vi "Create and Queue New Plugin Command.vi"(8 "error in (no error)":errorcluster, 9 "Matching Plugin":T1, 10 "New Plugin":T5, 11 "CIFPluginManager in":refnum<class "CIFPluginManager.lvclass">) -> (0 "error out":errorcluster)   [LabVIEW 2021, in "CIFPluginManager.lvclass"]
uses:
  CIFPluginManager.lvclass
  typedef/Plugin Load Command.ctl
  typedef/Loader Type.ctl
  typedef/Discovered Plugin.ctl
  <vilib>/CIF Foundation/CIF Core/CIFCore/Common/Typedef/Version.ctl
  typedef/Plugin Metadata.ctl
  CIFPluginManager.lvclass/CIFPluginManager.ctl
  typedef/Plugin Management Data.ctl
  <vilib>/gRPC/LabVIEW gRPC Library/Shared/grpcId.ctl
  gRPC/CIF_Manager_server/RPC Messages/cif_management_common_PluginStatusData.ctl
  gRPC/CIF_Manager_server/RPC Messages/cif_management_common_PluginStatusData_PluginState.ctl
  gRPC/CIF_Manager_server/RPC Messages/cif_management_common_TimingStatistics.ctl
  gRPC/CIF_Manager_server/RPC Messages/cif_common_TimingStats.ctl
  gRPC/CIF_Manager_server/RPC Messages/cif_management_common_FifoStatistics.ctl
  gRPC/CIF_Manager_server/RPC Messages/cif_management_common_Error.ctl
  gRPC/CIF_Manager_server/RPC Messages/cif_management_common_MonitorDoubles.ctl
  gRPC/CIF_Manager_server/RPC Messages/cif_management_common_MonitorU64.ctl
  gRPC/CIF_Manager_server/RPC Messages/cif_management_common_MonitorI64.ctl
  gRPC/CIF_Manager_server/RPC Messages/cif_management_common_Channels.ctl
  gRPC/CIF_Manager_server/RPC Messages/cif_management_common_Channel.ctl
  gRPC/CIF_Manager_server/RPC Messages/cif_management_common_ChannelDirection.ctl
  gRPC/CIF_Manager_server/RPC Messages/cif_management_common_ChannelPattern.ctl
  gRPC/CIF_Manager_server/CIF_Manager_server.lvlib
  <vilib>/CIF Foundation/CIF Core/CIFCore/Common/CIFCoreCommon.lvlib
  <vilib>/gRPC/LabVIEW gRPC Library/grpc-lvsupport-release.lvlib
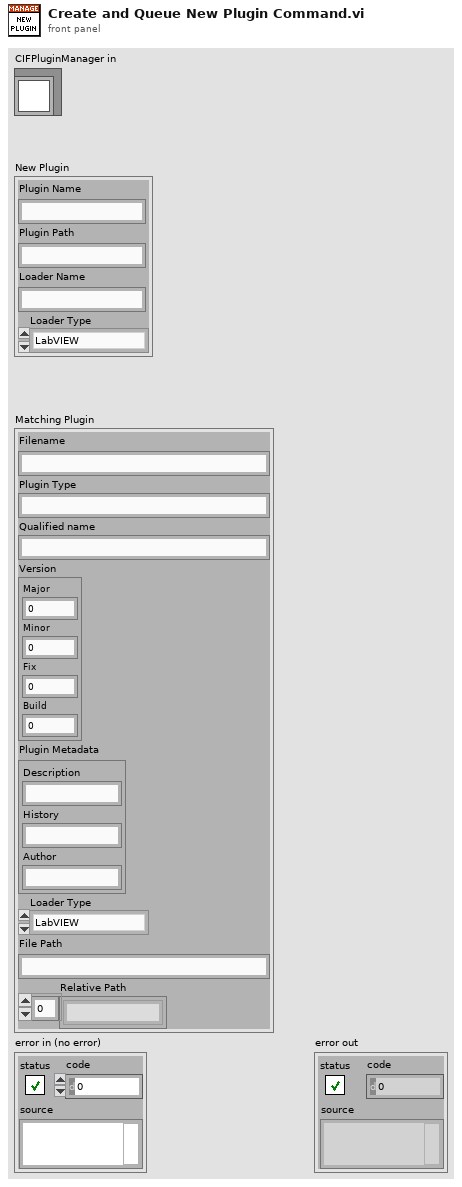
[diagram p1: front panel]
types:
  T1 = typedef "CIFPluginManager.lvclass/Discovered Plugin.ctl" = cluster{"Filename":string, "Plugin Type":string, "Qualified name":string, "Version":T2, "Plugin Metadata":T3, "Loader Type":T4, "File Path":string, "Relative Path":string[]}
  T2 = typedef "CIFCoreCommon.lvlib/Version.ctl" = cluster{"Major":i32, "Minor":i32, "Fix":i32, "Build":i32}
  T3 = typedef "CIFPluginManager.lvclass/Plugin Metadata.ctl" = cluster{"Description":string, "History":string, "Author":string}
  T4 = typedef "CIFPluginManager.lvclass/Loader Type.ctl" = enum16{"LabVIEW"}
  T5 = typedef "CIFPluginManager.lvclass/Plugin Load Command.ctl" = cluster{"Plugin Name":string, "Plugin Path":string, "Loader Name":string, "Loader Type":T4}
  T6 = typedef "CIFPluginManager.lvclass/Loader Map.ctl" = map{string, T7}
  T7 = typedef "CIFPluginManager.lvclass/Loaders.ctl" = cluster{"Loader Type":T4, "grpc_port":i32, "pid":u32, "gRPC ID":T8, "Load Timestamp":i64, "Unloading":bool, "Ready for removal":bool, "Unload Timestamp":i64}
  T8 = typedef "grpc-lvsupport-release.lvlib/grpcId.ctl" = u64
  T9 = typedef "CIFPluginManager.lvclass/Plugin Management Data.ctl" = cluster{"Unique Name":string, "Plugin Type":string, "gRPC Port":i32, "gRPC ID":T8, "Loader Type":T4, "Loader":string, "Version":T2, "Load Timestamp":i64, "Unload Timestamp":i64, "Unloading":bool, "Ready for removal":bool, "status":T10, "channels":T19}
  T10 = typedef "CIF_Manager_server.lvlib/cif_management_common_PluginStatusData.ctl" = cluster{"state":T11, "timing_statistics":T12, "fifo_statistics":T14, "error":T15, "monitor_doubles":T16, "monitor_u64s":T17, "monitor_i64s":T18}
  T11 = typedef "CIF_Manager_server.lvlib/cif_management_common_PluginStatusData_PluginState.ctl" = enum32{"PLUGINSTATE_UNKNOWN", "PLUGINSTATE_CREATING", "PLUGINSTATE_LISTENING", "PLUGINSTATE_RUNNING", "PLUGINSTATE_CLEANINGUP", "PLUGINSTATE_DESTROYING"}
  T12 = typedef "CIF_Manager_server.lvlib/cif_management_common_TimingStatistics.ctl" = cluster{"period":T13, "wake_error":T13, "execute":T13, "housekeep":T13, "idle":T13, "cleanup":T13, "custom_1":T13, "custom_2":T13}
  T13 = typedef "CIF_Manager_server.lvlib/cif_common_TimingStats.ctl" = cluster{"max":i64, "min":i64, "avg":dbl}
  T14 = typedef "CIF_Manager_server.lvlib/cif_management_common_FifoStatistics.ctl" = cluster{"from_t0":T13, "from_previous_plugin":T13, "output_error":T13}
  T15 = typedef "CIF_Manager_server.lvlib/cif_management_common_Error.ctl" = cluster{"status":bool, "code":i32}
  T16 = typedef "CIF_Manager_server.lvlib/cif_management_common_MonitorDoubles.ctl" = cluster{"double_1":dbl, "double_2":dbl, "double_3":dbl, "double_4":dbl}
  T17 = typedef "CIF_Manager_server.lvlib/cif_management_common_MonitorU64.ctl" = cluster{"u64_1":u64, "u64_2":u64, "u64_3":u64, "u64_4":u64}
  T18 = typedef "CIF_Manager_server.lvlib/cif_management_common_MonitorI64.ctl" = cluster{"i64_1":i64, "i64_2":i64, "i64_3":i64, "i64_4":i64}
  T19 = typedef "CIF_Manager_server.lvlib/cif_management_common_Channels.ctl" = cluster{"channels":T20[]}
  T20 = typedef "CIF_Manager_server.lvlib/cif_management_common_Channel.ctl" = cluster{"name":string, "direction":T21, "type":string, "custom_config":u8[], "connected":bool, "connected_name":string, "forced":bool, "channel_pattern":T22}
  T21 = typedef "CIF_Manager_server.lvlib/cif_management_common_ChannelDirection.ctl" = enum32{"CHANNELDIRECTION_UNKNOWN", "CHANNELDIRECTION_PUBLISHER", "CHANNELDIRECTION_SUBSCRIBER"}
  T22 = typedef "CIF_Manager_server.lvlib/cif_management_common_ChannelPattern.ctl" = enum32{"CHANNELPATTERN_UNKNOWN", "CHANNELPATTERN_TAG", "CHANNELPATTERN_FIFO", "CHANNELPATTERN_MULTIFIFO", "CHANNELPATTERN_BACKPRESSUREFIFO"}
  T23 = typedef "CIFPluginManager.lvclass/Plugin Management Data Map.ctl" = map{string, T9}
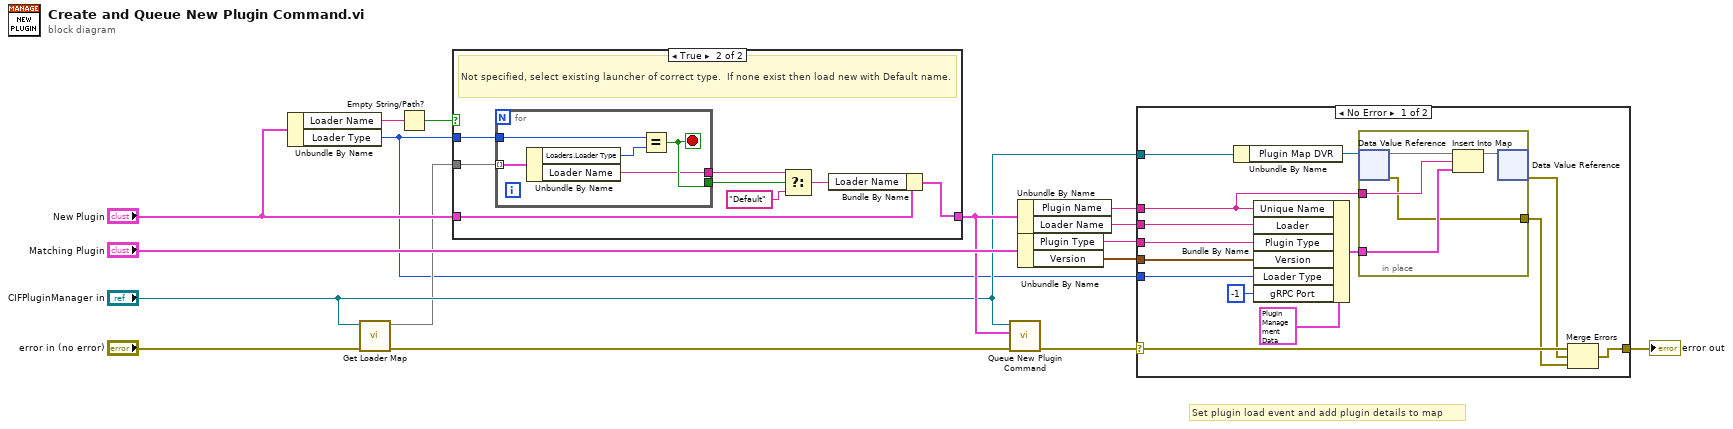
[diagram p0: block diagram]
diagram:
  # "Set plugin load event and add plugin details to map"
  n1 = Unbundle By Name("New Plugin") -> ("Loader Name"=w6:string, "Loader Type"=w1:T4)
  n2 = call "Get Loader Map.vi"("error in (no error)"="error in (no error)", "CIFPluginManager in"="CIFPluginManager in") -> ("error out"=w2:errorcluster, "Loader Map"=w4:T6)  [unwired: 8 in]
  n3 = Empty String/Path?(string/path=w6) -> (empty?=w9:bool)
  n4 = case shown="True" w9 {
    tunnel: "New Plugin" -> [w17 w22]
    tunnel: [w17 w20] -> w7
    tunnel: w1 -> [_ w25]
    tunnel: w4 -> [_ w18]
    frame False {
      # "When more loader types are supported add check to make sure type is correct"
      # "Launcher specified"
    }
    frame True {
      # "Not specified, select existing launcher of correct type.  If none exist then load new with Default name."
      n5 = for {
        tunnel: w18 -> [w30] mode=indexing
        tunnel: w25 -> [w29]
        tunnel: [w28] -> w24
        tunnel: [w27] -> w23
        stop <- w28 stop-if-true
        n6 = Unbundle By Name(w30) -> ("Loaders.Loader Type"=w26:T4, "Loader Name"=w27:string)
        n7 = Equal?(x=w29, y=w26) -> (x = y?=w28:bool)
      }
      n8 = Select(t=w23, s=w24, f="Default") -> (s? t:f=w21:string)
      n9 = Bundle By Name(cluster=w22, "Loader Name"=w21) -> (w20:T5)
    }
  }
  n10 = call "Queue New Plugin Command.vi"("error in (no error)"=w2, "New Plugin"=w7, "CIFPluginManager in"="CIFPluginManager in") -> ("error out"=w16:errorcluster)  [unwired: 8 in]
  n11 = Unbundle By Name(w7) -> ("Plugin Name"=w10:string, "Loader Name"=w15:string)
  n12 = Unbundle By Name("Matching Plugin") -> ("Plugin Type"=w13:string, "Version"=w12:T2)
  n13 = case shown="No Error" w16 {
    selector: w16 -> [w38 w50]
    tunnel: w15 -> [w34 _]
    tunnel: "CIFPluginManager in" -> [w40 _]
    tunnel: [w35 w50] -> w11
    tunnel: w13 -> [w43 _]
    tunnel: w12 -> [w41 _]
    tunnel: w10 -> [w33 _]
    tunnel: w1 -> [w31 _]
    frame No Error {
      n14 = Unbundle By Name(w40) -> ("Plugin Map DVR"=w39:refnum<data-value>)
      n15 = Bundle By Name(cluster=T9 {"Unique Name"="", "Plugin Type"="", "gRPC Port"=0, "gRPC ID"=0, "Loader Type"=enum."LabVIEW", "Loader"="", "Version"={"Major"=0, "Minor"=0, "Fix"=0, "Build"=0}, "Load Timestamp"=0, "Unload Timestamp"=0, "Unloading"=FALSE, "Ready for removal"=FALSE, "status"={"state"=enum."PLUGINSTATE_UNKNOWN", "timing_statistics"={"period"={"max"=0, "min"=0, "avg"=0.0}, "wake_error"={"max"=0, "min"=0, "avg"=0.0}, "execute"={"max"=0, "min"=0, "avg"=0.0}, "housekeep"={"max"=0, "min"=0, "avg"=0.0}, "idle"={"max"=0, "min"=0, "avg"=0.0}, "cleanup"={"max"=0, "min"=0, "avg"=0.0}, "custom_1"={"max"=0, "min"=0, "avg"=0.0}, "custom_2"={"max"=0, "min"=0, "avg"=0.0}}, "fifo_statistics"={"from_t0"={"max"=0, "min"=0, "avg"=0.0}, "from_previous_plugin"={"max"=0, "min"=0, "avg"=0.0}, "output_error"={"max"=0, "min"=0, "avg"=0.0}}, "error"={"status"=FALSE, "code"=0}, "monitor_doubles"={"double_1"=0.0, "double_2"=0.0, "double_3"=0.0, "double_4"=0.0}, "monitor_u64s"={"u64_1"=0, "u64_2"=0, "u64_3"=0, "u64_4"=0}, "monitor_i64s"={"i64_1"=0, "i64_2"=0, "i64_3"=0, "i64_4"=0}}, "channels"={"channels"=[]}} ("Plugin Management Data"), "Unique Name"=w33, "Loader"=w34, "Plugin Type"=w43, "Version"=w41, "Loader Type"=w31, "gRPC Port"=-1) -> (w42:T9)
      n16 = in-place {
        in-place-border: w33 -> [w49]
        in-place-border: w42 -> [w48]
        in-place-border: [w45] -> w37
        n17 = in-place-dvr #1(w39) -> (w47:T23, w45:errorcluster)
        n18 = Insert Into Map(map in=w47, key=w49, value=w48) -> (map out=w46:T23)  [unwired: 2 out]
        n19 = in-place-dvr #1(w46) -> (w36:errorcluster)  [unwired: 1 out]
      }
      n20 = Merge Errors(w38, w36, w37) -> (w35:errorcluster)
    }
    frame Error {
    }
  }
  "error out" <- w11
